vi "SwitchSolenoidValue.vi"(1 "Current Sole Value":enum16{""}(ring), 2 "Button":bool) -> (0 "New Sole Value":enum16{""}(ring))   [LabVIEW 2013]
uses:
  <vilib>/Rock Robotics/WPI/Solenoid/WPI_SolenoidValue.ctl
panel:
  # "Switch Value"
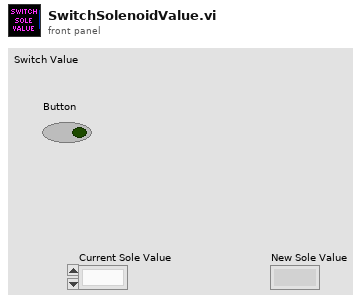
[diagram p1: front panel]
types:
  T1 = typedef "WPI_SolenoidValue.ctl" = enum16{"Off", "On", "Forward", "Reverse"}
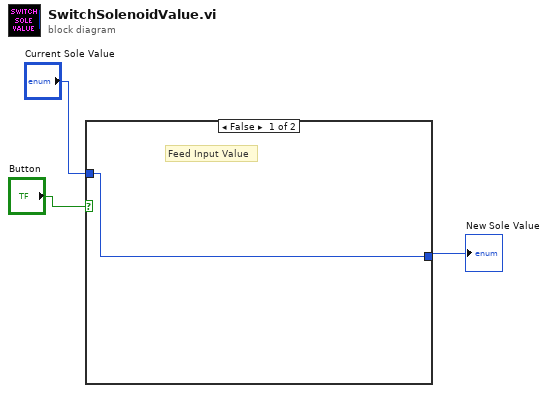
[diagram p0: block diagram]
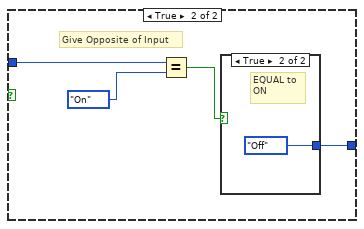
[diagram p2: hidden frame]
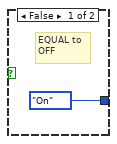
[diagram p3: hidden frame]
diagram:
  n1 = case shown="False" "Button" {
    tunnel: "Current Sole Value" -> [w4 w8]
    tunnel: [w4 w5] -> w1
    frame False {
      # "Feed Input Value"
    }
    frame True {
      # "Give Opposite of Input"
      n2 = Equal?(x=w8, y=WPI_SolenoidValue."On" ("Value")) -> (x = y?=w6:bool)
      n3 = case shown="True" w6 {
        tunnel: [WPI_SolenoidValue."On" ("Value") WPI_SolenoidValue."Off" ("Value")] -> w5
        frame False {
          # "EQUAL to\nOFF"
        }
        frame True {
          # "EQUAL to\nON"
        }
      }
    }
  }
  "New Sole Value" <- w1
